vi "Perform Action.vi"(8 "error in (no error)":errorcluster, 10 "Input":variant, 11 "Generate DC CFG in":refnum<class "Generate DC CFG.lvclass">) -> (0 "error out":errorcluster, 2 "Output":variant, 3 "Generate DC CFG out":refnum<class "Generate DC CFG.lvclass">)   [LabVIEW 2023, in "FGen Simulated CFGs.lvlib" / "Generate DC CFG.lvclass"]
uses:
  Generate DC CFG.lvclass
  Generate DC CFG.lvclass/Generate DC CFG.ctl
  FGen PXI/FGen PXI Std Waveform CFG/Std Waveform Action Pams.ctl
  FGen PXI/FGen PXI Std Waveform CFG/FGen PXI Std Waveform CFG.lvclass
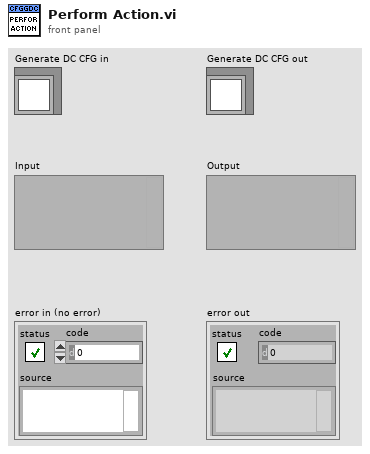
[diagram p1: front panel]
types:
  T1 = typedef "FGen PXI Std Waveform CFG.lvlib/FGen PXI Std Waveform CFG.lvclass/Std Waveform Action Pams.ctl" = cluster{"Frequency":dbl, "Amplitude":dbl, "DC Offset":dbl}
  T2 = cluster{"Channel":string, "Std Waveform Action Pams":T1}
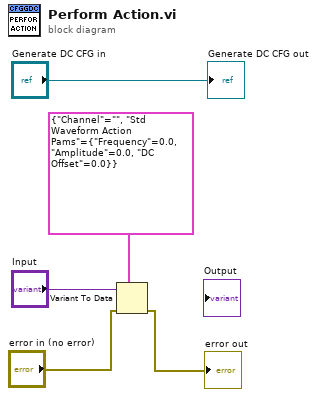
[diagram p0: block diagram]
diagram:
  n1 = Variant To Data(error in="error in (no error)", type=T2 {"Channel"="", "Std Waveform Action Pams"={"Frequency"=0.0, "Amplitude"=0.0, "DC Offset"=0.0}}, Variant="Input") -> (error out=→"error out":errorcluster)  [unwired: 1 out]
  "Generate DC CFG out" <- "Generate DC CFG in"
